vi "Configure Filter.vi"(8 "error in (no error)":errorcluster, 9 "Enable Digital Filter  (F: Disable)":bool, 10 "Channel (1: Channel 1)":u16(ring)=1 items=["Channel 1"=1, "Channel 2"=2, "Channel 3"=3, "Channel 4"=4], 11 "VISA resource name":refnum<visa-resource-name>) -> (0 "error out":errorcluster, 3 "VISA resource name out":refnum<visa-resource-name>)   [LabVIEW 2010, in "Agilent DSO1000 Series.lvlib"]
doc: "Configures the digitial filter setting for specific channel. Enable the filter to set it on."
uses:
  <instrlib>/Agilent DSO1000 Series/Agilent DSO1000 Series.lvlib
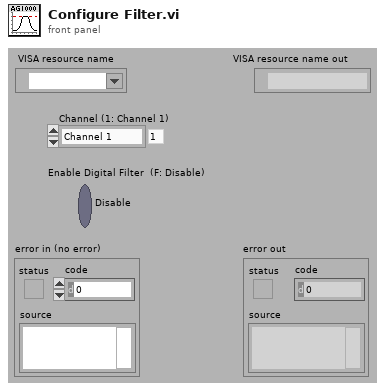
[diagram p1: front panel]
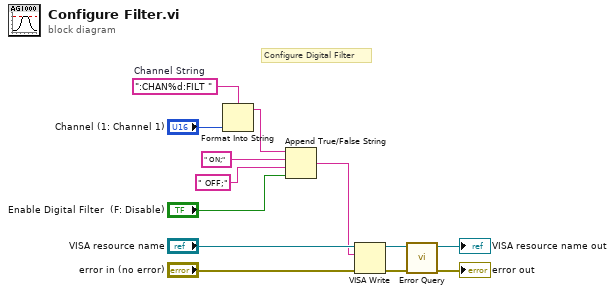
[diagram p0: block diagram]
diagram:
  w8 = ":CHAN%d:FILT "  # Channel String
  # "Configure Digital Filter"
  n1 = Format Into String(format string=w8, "Channel (1: Channel 1)") -> (resulting string=w5:string)  [unwired: 2 in, 1 out]
  n2 = Append True/False String(1:"Enable Digital Filter  (F: Disable)", 2:" OFF;", 3:" ON;" ("Digital Filter Command"), 4:w5) -> (0:w1:string)
  n3 = VISA Write(VISA resource name="VISA resource name", write buffer=w1, error in (no error)="error in (no error)") -> (VISA resource name out=w7:refnum<visa-resource-name>, error out=w6:errorcluster)  [unwired: 1 out]
  n4 = call <instrlib>:"Error Query.vi"("error in (no error)"=w6, "VISA resource name"=w7) -> ("error out"=→"error out":errorcluster, "VISA resource name out"=→"VISA resource name out":refnum<visa-resource-name>)  [unwired: 6 in, 2 out]
